vi "Value Change.vi"(5 "object ref in":T2, 8 "error in (no error)":errorcluster, 9 "old values":string[][](array[string]), 10 "Cluster":T1, 11 "List Box Enum Column in":refnum<class "List Box Enum Column.lvclass">) -> (0 "error out":errorcluster, 3 "List Box Enum Column out":refnum<class "List Box Enum Column.lvclass">)   [LabVIEW 2013, in "Table Manager.lvlib" / "List Box Enum Column.lvclass"]
uses:
  List Box Enum Column.lvclass
  TagSelectModule/Source/editor node/object ref.ctl
  <vilib>/NI/Tag Bus Data Framework/Configuration Editor/Classes/Engine Parent/Engine Parent Editor Node.lvclass
  <vilib>/NI/Tag Bus Data Framework/Configuration Editor/Classes/Module editor node/module editor node.lvclass
  Table Manager/Cell Change.ctl
  Column/Column.lvclass/Column.ctl
  Column/Read Call Back VI.vi
  TagSelectModule/Source/editor node/tag select module editor node.lvclass
  Table Manager.lvlib
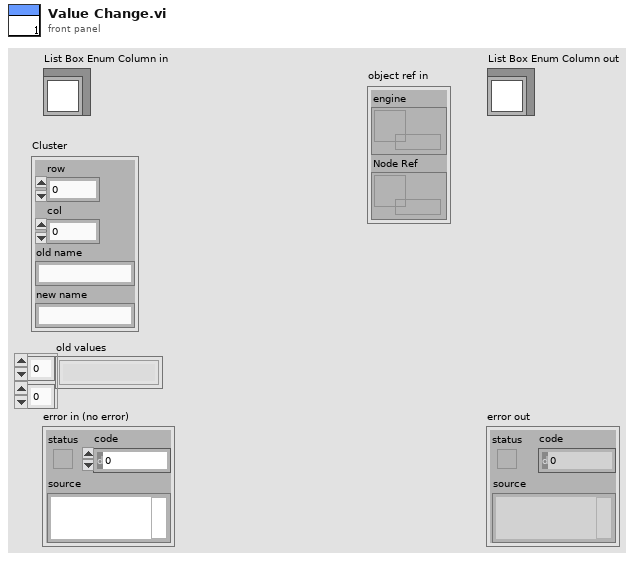
[diagram p1: front panel]
types:
  T1 = typedef "Table Manager.lvlib/Cell Change.ctl" = cluster{"row":i32, "col":i32, "old name":string, "new name":string}
  T2 = typedef "tag select module editor node.lvclass/object ref.ctl" = cluster{"engine":refnum<data-value>, "Node Ref":refnum<data-value>}
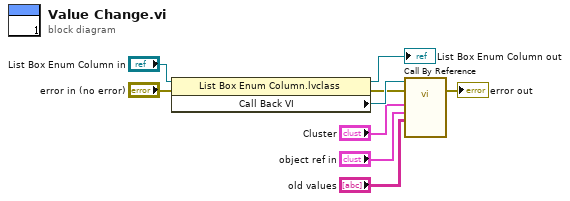
[diagram p0: block diagram]
diagram:
  n1 = property class="List Box Enum Column.lvclass"(reference="List Box Enum Column in", error in="error in (no error)") -> (reference out=→"List Box Enum Column out":refnum<class "List Box Enum Column.lvclass">, error out=w7:errorcluster, "Call Back VI"=w9:refnum<vi>)
  n2 = call-by-ref "?"(reference=w9, error in=w7, "old values"="old values", "object ref in"="object ref in", "Cluster"="Cluster") -> (error out=→"error out":errorcluster)  [unwired: 8 in, 2 out]
